vi "PNA_SMC_SET-CWFREQ.vi"(0 "Session In":refnum<visa-resource-name>="TCPIP0::K-Instr0000.local::hislip0::INSTR", 5 "error in":errorcluster {"code" format="%.0x"}, 7 "FREQ":dbl=20.0 format="%#_6f", 8 "Timeout":u32=5000, 9 "Units":i64(ring)=1000000000 items=["GHz"=1000000000, "MHZ"=1000000], 10 "RO(T)":bool, 11 "CH":i32=3, 13 "Source":i32=1) -> (12 "freq":dbl=5.0, 14 "Session Out":refnum<visa-resource-name>="TCPIP0::K-Instr0000.local::hislip0::INSTR", 19 "error out":errorcluster {"code" format="%.0x"})   [LabVIEW 2018]
doc: "Applicable Models: All with Spectrum Analysis Options (S9x09xxA/B, S9x09xA/B)\n\n(Read-Write) Set and read the source CW frequency.\n \nParameters\n \n \n<ch>\n Any existing SA channel. If unspecified, value is set to 1.\n \n<port>\n Source port number of the VNA. If unspecified, value is set to 1. To make settings for ports that are not simple numbers, use the [src] argument.\n \n<num>\n CW frequency in Hz. Choose a value within the frequency range of the analyzer.\n \n[,src]\n String. (NOT case sensitive). Source port. Optional. Use SOUR:CAT? to return a list of valid port names.\n\nWhile this argument can be used to make settings for ALL ports, it is designed to access ports such as an external source, or one of the Source 2 outputs on the 2-port 2-source PNA-X model such as \"Port 1 Src2\". Otherwise, the <port> argument performs the same function. If both arguments are specified, [src] takes priority.\n \nExamples\n SENS:SA:SOUR:FREQ:CW 1e10\n\nsense2:sa:source:frequency:cw 1e9,\"Port 1 Src2\"\n \nQuery Syntax\n SENSe<ch>:SA:SOURce<port>:FREQuency:CW?\n \nReturn Type\n Numeric\n \nDefault\n Center frequency of the analyzer"
uses:
  lib functions/Agilent ENA Series.lvlib
panel:
  out "concatenated string":string="sens3:sa:sour1:freq:cw?\nsens3:sa:sour1:freq:cw 5000000000.000000\n"
  # "Instrument Address"
  # "Select Source"
  # "Conditions"
  # "Is Read Only (T)"
  # "Channel"
  # "Source"
  # "Inst Timeout(ms)"
  # "Set Freq"
  # "Freq"
  # "Read"
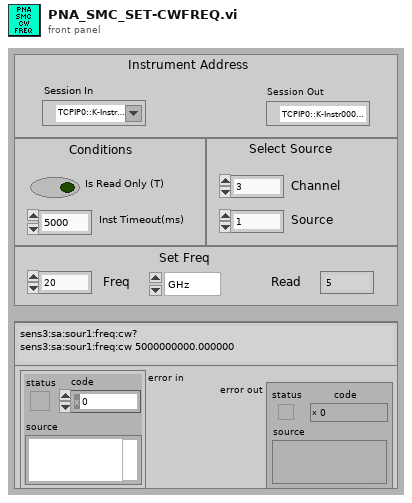
[diagram p1: front panel]
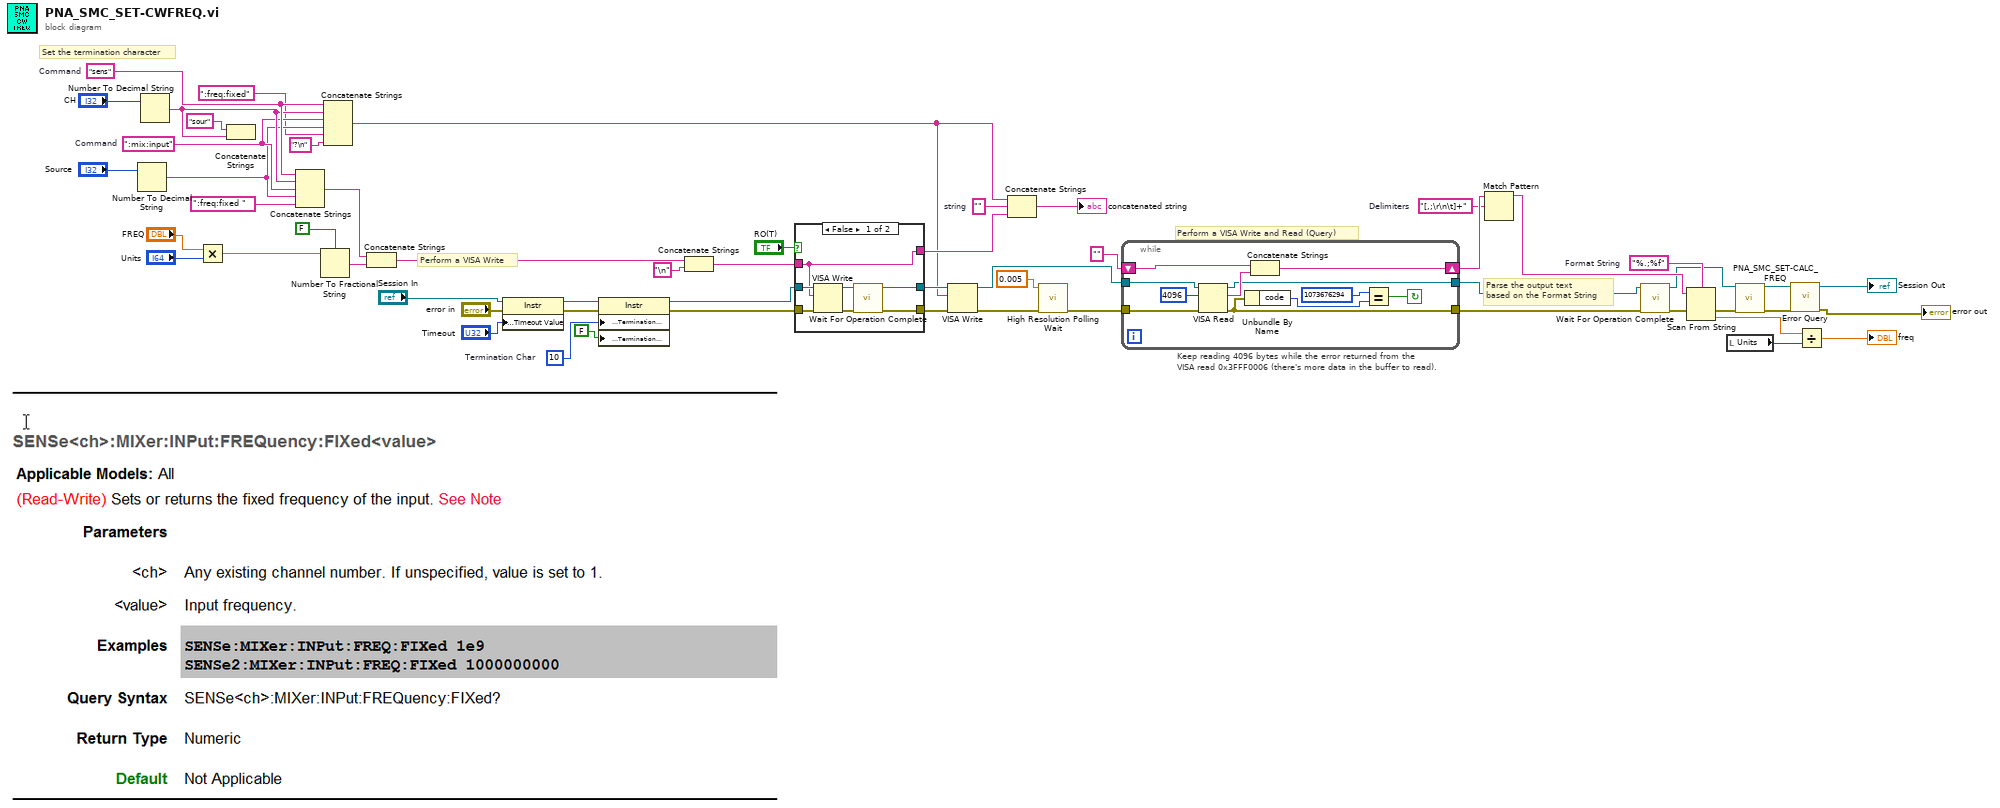
[diagram p0: block diagram]
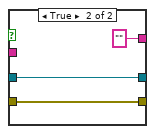
[diagram p2: hidden frame]
diagram:
  w25 = ":mix:input"  # Command
  w31 = ""  # string
  w36 = "[,;\r\n\t]+"  # Delimiters
  w37 = "%.;%f"  # Format String
  w27 = "sens"  # Command
  w48 = u8 10  # Termination Char
  # "Parse the output text based on the Format String"
  # "Perform a VISA Write and Read (Query)"
  # "Keep reading 4096 bytes while the error returned from the\nVISA read 0x3FFF0006 (there's more data in the buffer to read)."
  # "Perform a VISA Write"
  # "Set the termination character"
  n1 = Number To Decimal String(number="Source") -> (decimal integer string=w24:string)  [unwired: 1 out]
  n2 = Number To Decimal String(number="CH") -> (decimal integer string=w26:string)  [unwired: 1 out]
  n3 = Multiply(x="FREQ", y="Units") -> (x*y=w21:dbl)
  n4 = Concatenate Strings("sour" ("staticText"), w26) -> ()  [unwired: 1 out]
  n5 = Concatenate Strings(w27, w26, w25, w24, ":freq:fixed " ("Command")) -> (w22:string)
  n6 = Number To Fractional String(use system decimal point (T)=FALSE, number=w21) -> (F-format string=w19:string)  [unwired: 2 in]
  n7 = Concatenate Strings(w27, w26, w25, w24, ":freq:fixed" ("Command"), "?\n" ("Command")) -> (w14:string)
  n8 = Concatenate Strings(w22, w19) -> (w42:string)
  n9 = property class="Instr"(reference="Session In", error in="error in", "General Settings:Timeout Value"="Timeout") -> (reference out=w47:refnum<visa-resource-name>, error out=w50:errorcluster)
  n10 = property class="Instr"(reference=w47, error in=w50, "Message Based Settings:Termination Character"=w48, "Message Based Settings:Termination Character Enable"=FALSE ("enable")) -> (reference out=w35:refnum<visa-resource-name>, error out=w49:errorcluster)
  n11 = Concatenate Strings(w42, "\n" ("StaticText")) -> (w43:string)
  n12 = case shown="False" "RO(T)" {
    tunnel: w49 -> [w63 w65]
    tunnel: [w60 w65] -> w44
    tunnel: w43 -> [w61 _]
    tunnel: w35 -> [w62 w66]
    tunnel: [w57 w66] -> w34
    tunnel: [w61 ""] -> w15
    frame False {
      n13 = VISA Write(VISA resource name=w62, write buffer=w61, error in (no error)=w63) -> (VISA resource name out=w58:refnum<visa-resource-name>, error out=w59:errorcluster)  [unwired: 1 out]
      n14 = call "Wait For Operation Complete.vi"("error in (no error)"=w59, "VISA resource name"=w58) -> ("error out"=w60:errorcluster, "VISA resource name out"=w57:refnum<visa-resource-name>)  [unwired: 8 in]
    }
    frame True {
    }
  }
  n15 = VISA Write(VISA resource name=w34, write buffer=w14, error in (no error)=w44) -> (VISA resource name out=w11:refnum<visa-resource-name>, error out=w12:errorcluster)  [unwired: 1 out]
  n16 = Concatenate Strings(w14, w31, w15) -> (→"concatenated string":string)
  n17 = call <vilib>:"High Resolution Polling Wait.vi"("error in (no error)"=w12, "seconds to wait"=0.005) -> ("error out"=w13:errorcluster)  [unwired: 9 in]
  n18 = while {
    tunnel: w11 -> [w74]
    shift-right: [w68] -> w39
    shift-left: "" -> [w73]
    tunnel: w13 -> [w71]
    tunnel: [w70] -> w7
    tunnel: [w67] -> w8
    stop <- w69 continue-if-true
    n19 = VISA Read(VISA resource name=w74, byte count=u32 4096 ("byte count (0)"), error in (no error)=w71) -> (VISA resource name out=w67:refnum<visa-resource-name>, read buffer=w72:string, error out=w70:errorcluster)  [unwired: 1 out]
    n20 = Unbundle By Name(w70) -> ("code"=w76:i32)
    n21 = Concatenate Strings(w73, w72) -> (w68:string)
    n22 = Equal?(x=1073676294, y=w76) -> (x = y?=w69:bool)
  }
  n23 = Match Pattern(string=w39, regular expression=w36) -> (before substring=w38:string)  [unwired: 1 in, 3 out]
  n24 = call "Wait For Operation Complete.vi"("error in (no error)"=w7, "VISA resource name"=w8) -> ("error out"=w6:errorcluster, "VISA resource name out"=w9:refnum<visa-resource-name>)  [unwired: 8 in]
  n25 = Scan From String(format string=w37, input string=w38, error in=w6) -> (error out=w5:errorcluster, output 1=w29:dbl)  [unwired: 2 in, 2 out]
  n26 = local read "Units"() -> (w16:i64)
  n27 = call "PNA_SMC_SET-CALC_FREQ.vi"("Session In"=w9, "error in"=w5) -> ("Session Out"=w3:refnum<visa-resource-name>, "error out"=w4:errorcluster)  [unwired: 12 in]
  n28 = call "Error Query.vi"("error in (no error)"=w4, "VISA resource name"=w3) -> ("error out"=→"error out":errorcluster, "VISA resource name out"=→"Session Out":refnum<visa-resource-name>)  [unwired: 6 in, 2 out]
  n29 = Divide(x=w29, y=w16) -> (x/y=→"freq":dbl)
